vi "raw data manage.vi"() -> ()   [LabVIEW 2019]
uses:
  Display/Public/Controls/RGB Gains.ctl
  Display/Display.lvclass
panel:
  in  "Matrix":u32[][](array[colorbox])
  in  "Number of panels":i32
  in  "Accessors:RGB Gains":T1
  out "Array":u8[](array[numeric])
  out "Matrix 2":u32[][](array[colorbox])
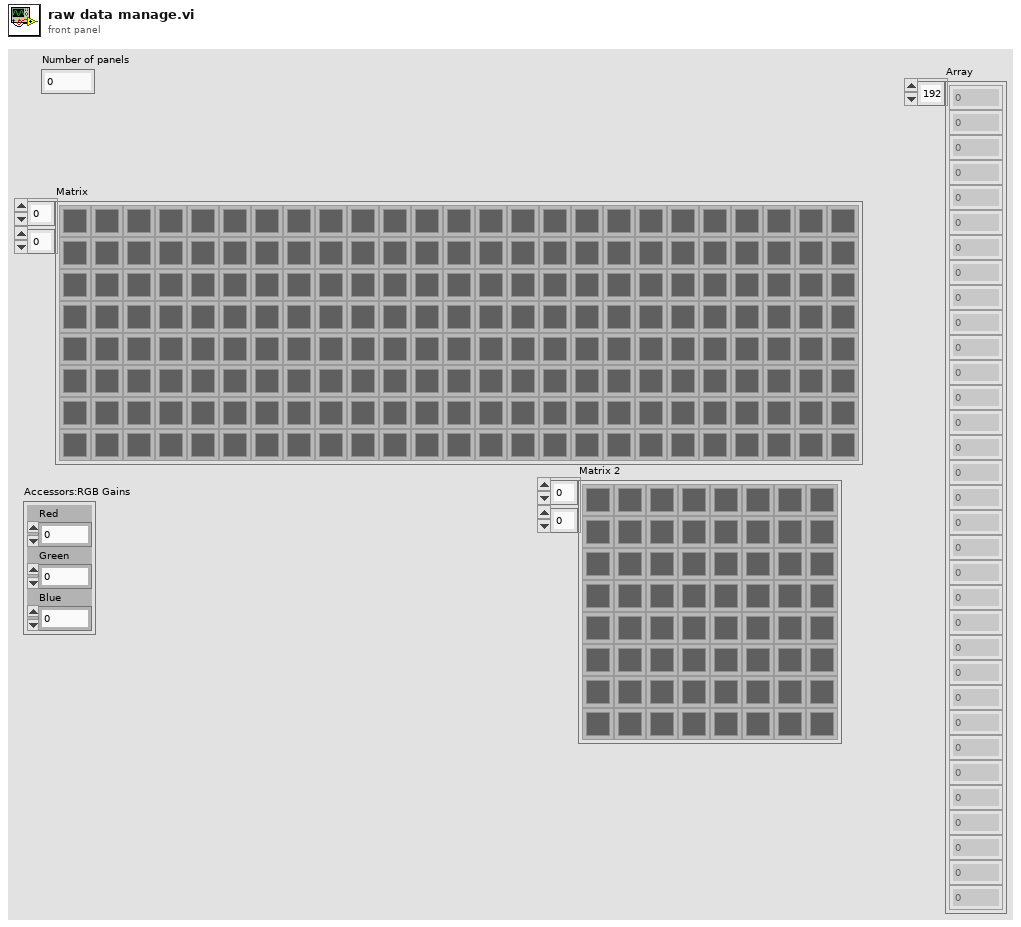
[diagram p1: front panel]
types:
  T1 = typedef "Display.lvclass/RGB Gains.ctl" = cluster{"Red":sgl, "Green":sgl, "Blue":sgl}
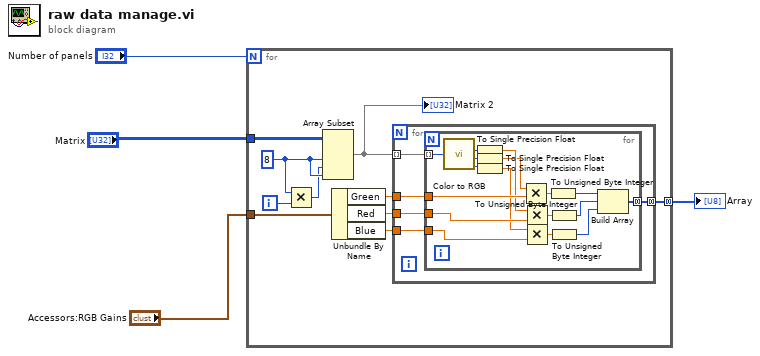
[diagram p0: block diagram]
diagram:
  n1 = for {
    N: "Number of panels" -> [_]
    tunnel: "Matrix" -> [w14]
    tunnel: "Accessors:RGB Gains" -> [w11]
    tunnel: [w7] -> w4 mode=concatenating
    i -> [w13]
    w12 = 8 ("length")
    n2 = Multiply(x=w12, y=w13) -> (x*y=w6:i32)
    n3 = Array Subset(array=w14, length (row)=w12, index (col)=w6, length (col)=w12) -> (w5:u32[][])  [unwired: 1 in]
    "Matrix 2" <- w5
    n4 = Unbundle By Name(w11) -> ("Green"=w10:sgl, "Red"=w9:sgl, "Blue"=w8:sgl)
    n5 = for {
      tunnel: w5 -> [w19] mode=indexing
      tunnel: [w18] -> w7 mode=concatenating
      tunnel: w10 -> [w17]
      tunnel: w9 -> [w16]
      tunnel: w8 -> [w15]
      n6 = for {
        tunnel: w19 -> [w36] mode=indexing
        tunnel: [w35] -> w18 mode=concatenating
        tunnel: w17 -> [w29]
        tunnel: w16 -> [w28]
        tunnel: w15 -> [w27]
        n7 = call <vilib>:"Color to RGB.vi"("Color"=w36) -> ("R"=w26:u8, "G"=w24:u8, "B"=w22:u8)  [unwired: 1 out]
        n8 = To Single Precision Float(number=w26) -> (single precision float=w25:sgl)
        n9 = To Single Precision Float(number=w24) -> (single precision float=w23:sgl)
        n10 = To Single Precision Float(number=w22) -> (single precision float=w21:sgl)
        n11 = Multiply(x=w23, y=w29) -> (x*y=w34:sgl)
        n12 = Multiply(x=w25, y=w28) -> (x*y=w32:sgl)
        n13 = Multiply(x=w21, y=w27) -> (x*y=w20:sgl)
        n14 = To Unsigned Byte Integer(number=w34) -> (unsigned 8bit integer=w33:u8)
        n15 = To Unsigned Byte Integer(number=w32) -> (unsigned 8bit integer=w31:u8)
        n16 = To Unsigned Byte Integer(number=w20) -> (unsigned 8bit integer=w30:u8)
        n17 = Build Array(w33, w31, w30) -> (w35:u8[])
      }
    }
  }
  "Array" <- w4
